vi "Main Recipe.vi"() -> ()   [LabVIEW 2011]
uses:
  System.Windows.Forms
panel:
  in  "stop":bool
  in  "Step Name":string
  in  "Delay":dbl
  in  "Ramp":dbl
  in  "Time":dbl
  in  "Tab Control":enum32{"Steps", "XML", "Valves", "MFC", "PC"}(tab)
  in  "Steps":i32(listbox)
  out "XML":refnum<k24>(container)
  in  "Valves":T1(array[cluster])
  in  "MFCs":T2(array[cluster])
  in  "Add Step":bool
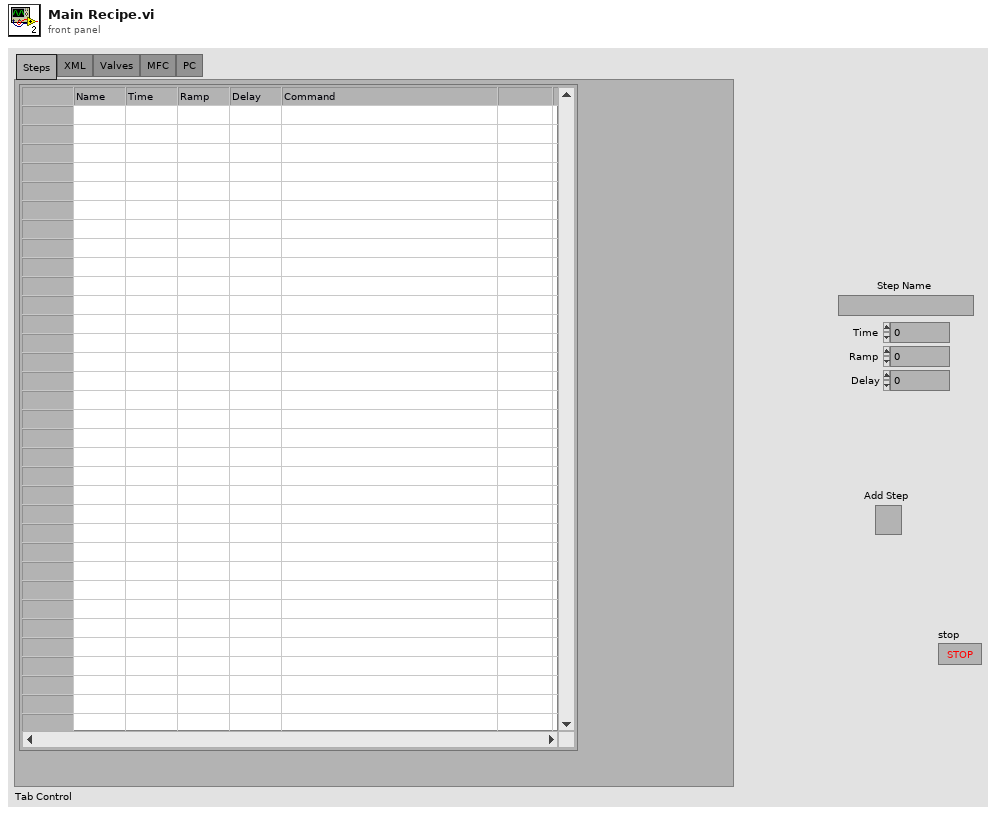
[diagram p1: front panel]
types:
  T1 = cluster{"Index":dbl, "Enabled":bool, "Value":bool}[][]
  T2 = cluster{"Enabled":bool, "Index 2":dbl, "Value":dbl}[][]
  T3 = cluster{"Valve":i32, "Enabled":bool, "Value":bool}
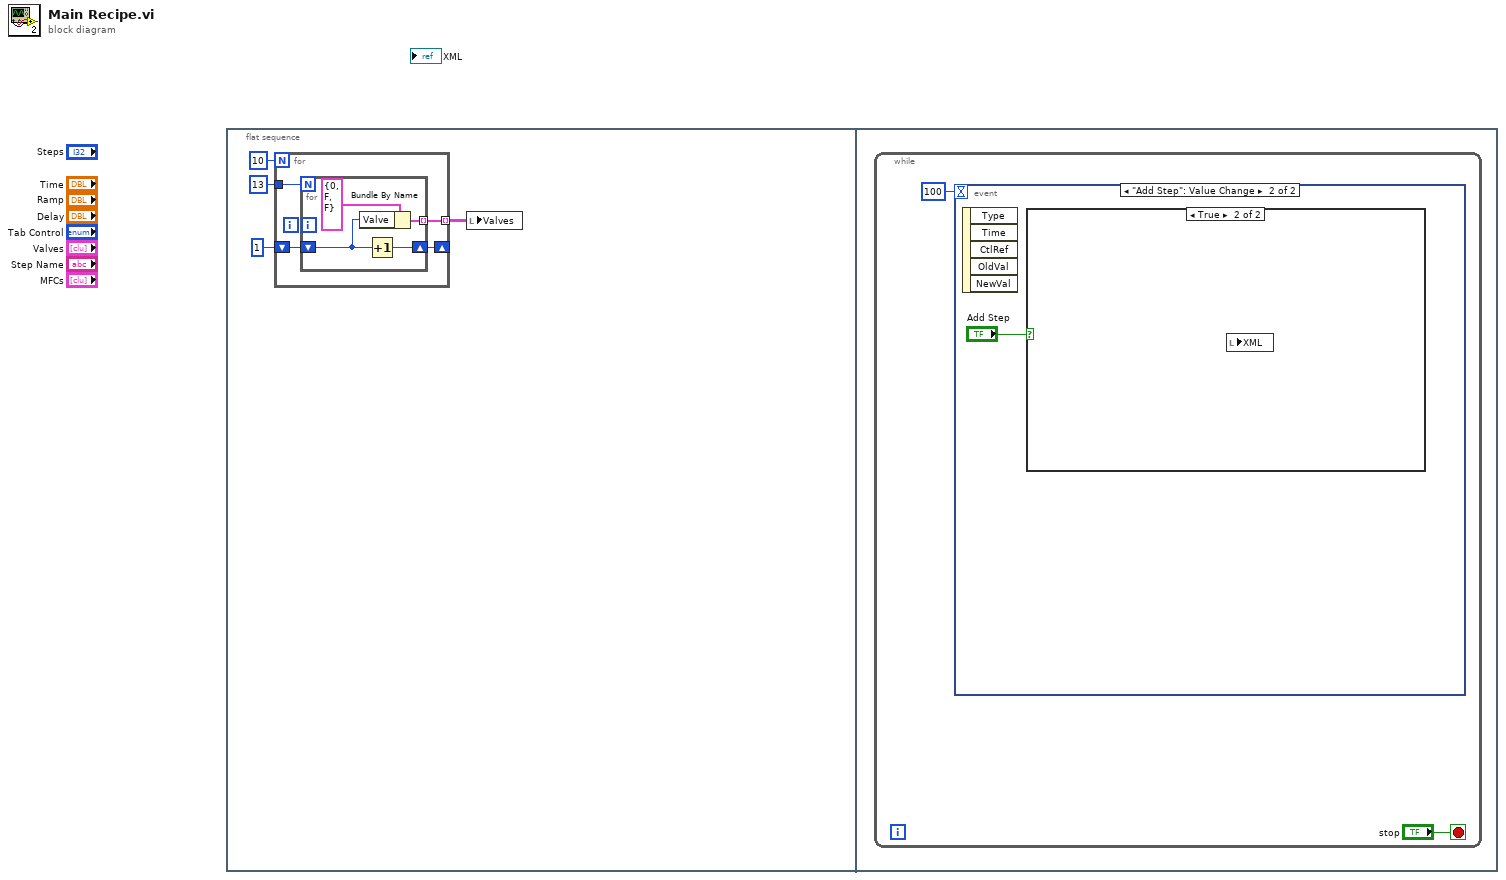
[diagram p0: block diagram]
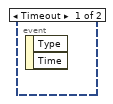
[diagram p2: hidden frame]
diagram:
  n1 = flat-sequence {
    frame #0 {
      n2 = for {
        N: 10 ("dimension size") -> [_]
        tunnel: 13 ("dimension size") -> [w8]
        tunnel: [w7] -> w3 mode=indexing
        shift-right: [w5] -> _
        shift-left: 1 -> [w6]
        n3 = for {
          N: w8 -> [_]
          tunnel: [w12] -> w7 mode=indexing
          shift-right: [w10] -> w5
          shift-left: w6 -> [w9]
          n4 = Bundle By Name(cluster=T3 {"Valve"=0, "Enabled"=FALSE, "Value"=FALSE} ("Cluster"), "Valve"=w9) -> (w12:T3)
          n5 = Increment(x=w9) -> (x+1=w10:i32)
        }
      }
      n6 = local write "Valves"(w3) -> ()
    }
    frame #1 {
      n7 = while {
        stop <- "stop" stop-if-true
        n8 = event shown="[1] \"Add Step\": Value Change" {
          selector: _ -> [_ _]
          dyn-events: _ -> [_ _]
          timeout: 100 -> [_ _]
          event Timeout {
            n9 = event-data() -> ()  [unwired: 1 in, 2 out]
          }
          event "Add Step": Value Change {
            n10 = event-data() -> ()  [unwired: 1 in, 5 out]
            n11 = case shown="True" "Add Step" {
              frame False {
              }
              frame True {
                n12 = local read "XML"() -> ()  [unwired: 1 in]
              }
            }
          }
        }
      }
    }
  }
